vi "check_sum.vi"() -> ()   [LabVIEW 2015]
panel:
  out "배열 2":string[][](array[string])
  in  "배열":string[](array[string])
  out "count":i32
  out "Error Out":errorcluster caption="에러 출력"
  in  "Error In":errorcluster caption="에러 입력"
  out "2진수":u32 format="%b"
  in  "16진수 문자열":string
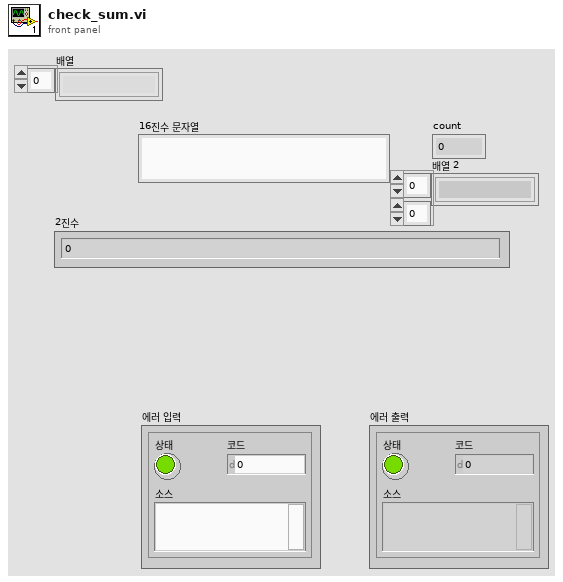
[diagram p1: front panel]
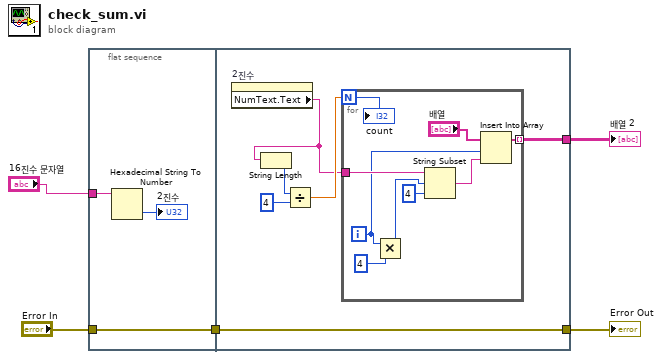
[diagram p0: block diagram]
diagram:
  n1 = flat-sequence {
    tunnel: [w7] -> w5
    tunnel: "Error In" -> [w7]
    tunnel: "16진수 문자열" -> [w6]
    tunnel: w5 -> [w14]
    tunnel: [w14] -> w3
    tunnel: [w9] -> w1
    frame #0 {
      n2 = Hexadecimal String To Number(string=w6) -> (number=→"2진수":u32)  [unwired: 2 in, 1 out]
    }
    frame #1 {
      n3 = property on="2진수" class="DigNum (엄격한)"() -> ("NumText.Text"=w10:string)  [unwired: 2 in, 2 out]
      n4 = String Length(string=w10) -> (length=w13:i32)
      n5 = Divide(x=w13, y=4) -> (x/y=w11:dbl)
      n6 = for {
        N: w11 -> [w19]
        tunnel: w10 -> [w20]
        tunnel: [w16] -> w9 mode=indexing
        i -> [w15]
        n7 = Multiply(x=w15, y=4) -> (x*y=w21:i32)
        n8 = String Subset(string=w20, offset (0)=w21, length (rest)=4 ("길이(나머지)")) -> (substring=w18:string)
        n9 = Insert Into Array(array="배열", index=w15, new element=w18) -> (w16:string[])
        "count" <- w19
      }
    }
  }
  "Error Out" <- w3
  "배열 2" <- w1
